vi "SetCursorMode.vi"(10 "Visible":bool, 11 "Graph Refnum":refnum<vi>) -> (3 "Graph Refnum 2":refnum<vi>)   [LabVIEW 2013, in "main.lvlib"]
uses:
  main.lvlib
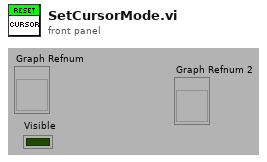
[diagram p1: front panel]
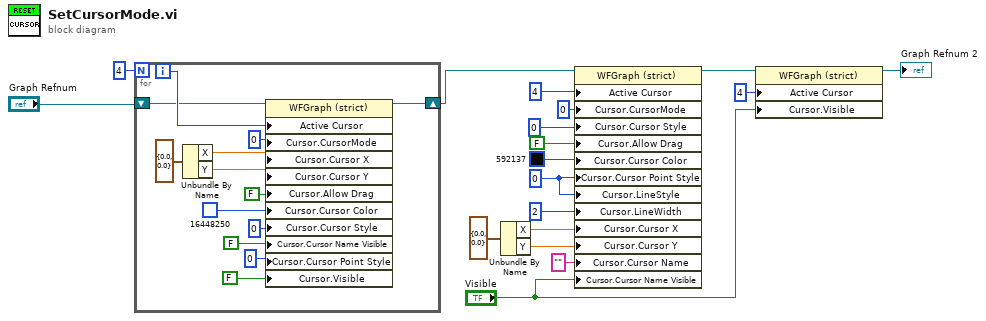
[diagram p0: block diagram]
diagram:
  w9 = u8 0 ("Cursor.Cursor Point Style")
  n1 = for {
    N: 4 -> [_]
    shift-right: [w20] -> w11
    shift-left: "Graph Refnum" -> [w19]
    i -> [w22]
    n2 = Unbundle By Name(cluster{"X":dbl, "Y":dbl} {"X"=0.0, "Y"=0.0} ("input cluster")) -> ("X"=w30:dbl, "Y"=w29:dbl)
    n3 = property class="WFGraph (strict)"(reference=w19, "Active Cursor"=w22, "Cursor.CursorMode"=u32 0 ("Cursor.Cursor Mode"), "Cursor.Cursor X"=w30, "Cursor.Cursor Y"=w29, "Cursor.Allow Drag"=FALSE, "Cursor.Cursor Color"=u32 16448250, "Cursor.Cursor Style"=u8 0, "Cursor.Cursor Name Visible"=FALSE, "Cursor.Cursor Point Style"=0, "Cursor.Visible"=FALSE) -> (reference out=w20:refnum<vi>)  [unwired: 1 in, 1 out]
  }
  n4 = Unbundle By Name(cluster{"X":dbl, "Y":dbl} {"X"=0.0, "Y"=0.0} ("input cluster")) -> ("X"=w8:dbl, "Y"=w7:dbl)
  n5 = property class="WFGraph (strict)"(reference=w11, "Active Cursor"=u32 4, "Cursor.CursorMode"=u32 0 ("Cursor.Cursor Mode"), "Cursor.Cursor Style"=u8 0, "Cursor.Allow Drag"=FALSE, "Cursor.Cursor Color"=u32 592137, "Cursor.Cursor Point Style"=w9, "Cursor.LineStyle"=w9, "Cursor.LineWidth"=u8 2 ("Cursor.Line Width"), "Cursor.Cursor X"=w8, "Cursor.Cursor Y"=w7, "Cursor.Cursor Name"="", "Cursor.Cursor Name Visible"="Visible") -> (reference out=w4:refnum<vi>)  [unwired: 1 in, 1 out]
  n6 = property class="WFGraph (strict)"(reference=w4, "Active Cursor"=u32 4, "Cursor.Visible"="Visible") -> (reference out=→"Graph Refnum 2":refnum<vi>)  [unwired: 1 in, 1 out]
